vi "Compile Event Measure 1.1 Data.vi"(7 "RIO Address":string, 8 "error in (no error)":errorcluster, 11 "Device Item Ref in":T3 format="%.0x") -> (0 "error out":errorcluster, 2 "Event Timing Measures":T1[](array[typedef]), 3 "Device Item Ref out":T3 format="%.0x")   [LabVIEW 2015, in "Engine Simulation Toolkit System Explorer.lvlib"]
uses:
  Engine Simulation Toolkit System Explorer.lvlib
  <vilib>/NI Veristand/Custom Device API/Custom Device Item Ref.ctl
  Shared/1.1 Event Timing Measure Engine Data.ctl
  Shared/1.0 Event Timing Measure FIFO Idxs.ctl
  Polarity.ctl
  Shared/Constants and GUIDs.vi
  <vilib>/NI Veristand/Custom Device Tools/Custom Device Utility Library/NI VeriStand - Search for All Items by GUID.vi
  Shared/Engine Simulation Toolkit Shared.lvlib
  <vilib>/NI VeriStand/Custom Device Tools/Custom Device Utility Library/Custom Device Utility Library.lvlib
  <vilib>/NI VeriStand/Custom Device API/Custom Device API.lvlib
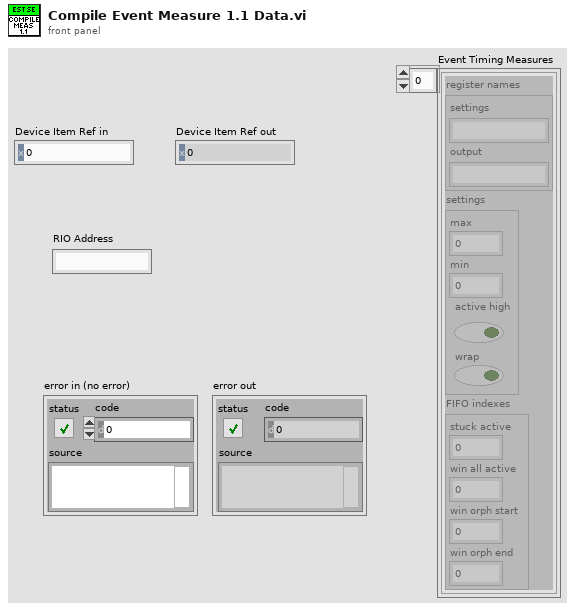
[diagram p1: front panel]
types:
  T1 = typedef "Engine Simulation Toolkit Shared.lvlib/1.1 Event Timing Measure Engine Data.ctl" = cluster{"register names":cluster{"settings":string, "output":string}, "settings":cluster{"max":u16, "min":u16, "active high":bool, "wrap":bool}, "FIFO indexes":T2}
  T2 = typedef "Engine Simulation Toolkit Shared.lvlib/1.0 Event Timing Measure FIFO Idxs.ctl" = cluster{"stuck active":i32, "win all active":i32, "win orph start":i32, "win orph end":i32}
  T3 = typedef "Custom Device API.lvlib/Custom Device Item Ref.ctl" = u64
  T4 = typedef "Engine Simulation Toolkit Shared.lvlib/Channel.ctl" = cluster{"Name":string, "Units":string, "Default":dbl, "Description":string, "Scalable":bool}
  T5 = typedef "Custom Device API.lvlib/Custom Device Item Info.ctl" = cluster{"Name":string, "Is Channel":bool, "GUID":string, "Is Waveform":bool}
  T6 = typedef "Engine Simulation Toolkit System Explorer.lvlib/Event Timing Window.ctl" = cluster{"Name":string, "Min":dbl, "Max":dbl, "Ref":dbl}
  T7 = typedef "Engine Simulation Toolkit System Explorer.lvlib/Event Timing Measurement.ctl" = cluster{"Name":string, "Bitfile name":string, "Window":string, "Polarity":T8}
  T8 = typedef "Engine Simulation Toolkit System Explorer.lvlib/Polarity.ctl" = enum16{"Active low", "Active high"}
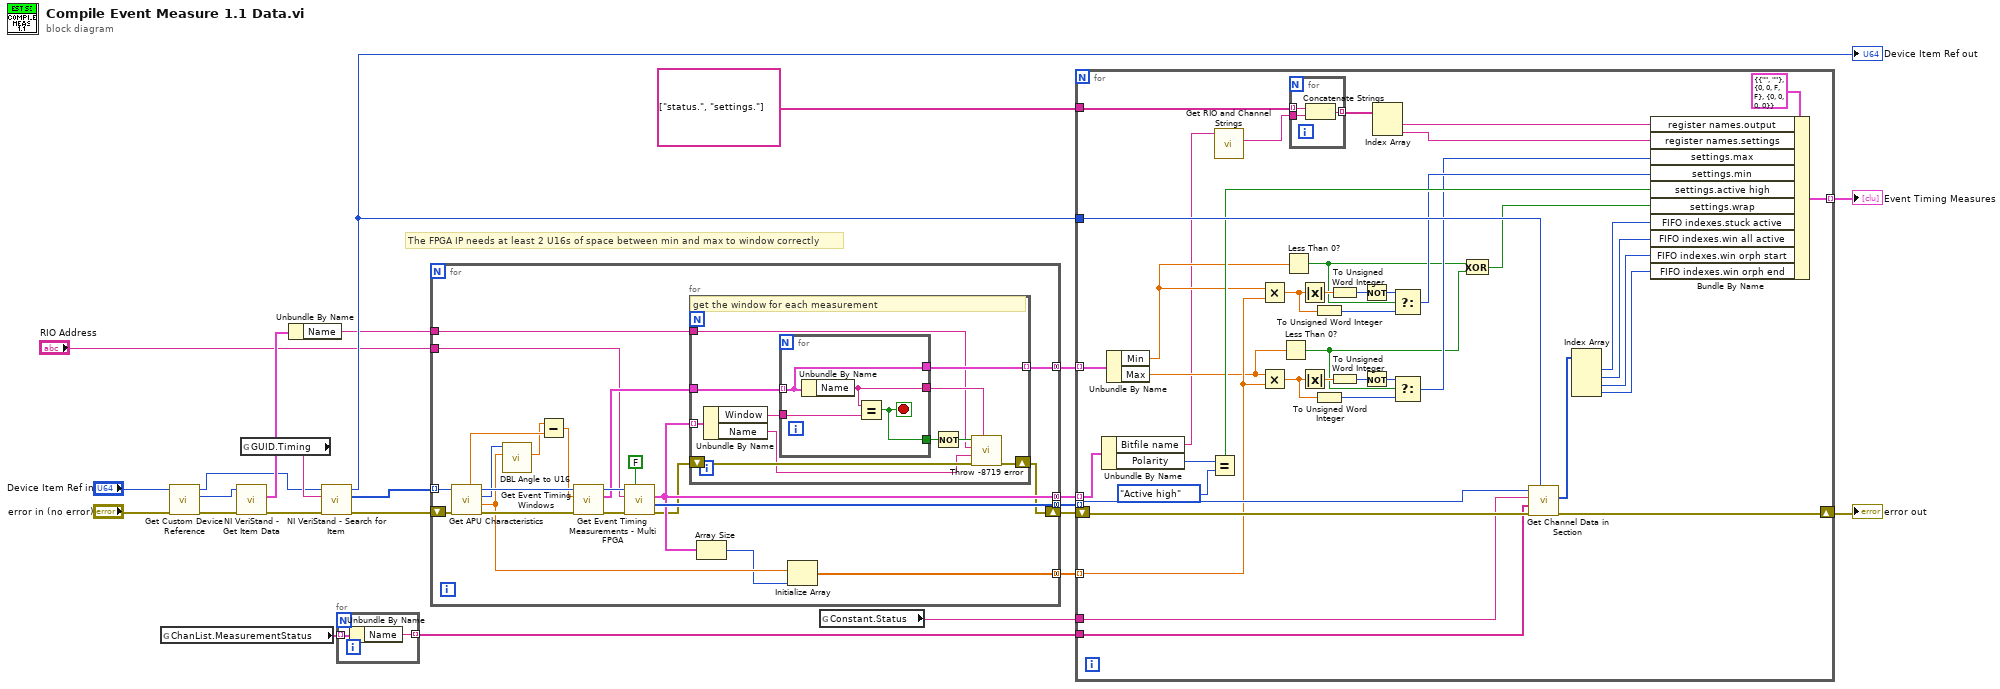
[diagram p0: block diagram]
diagram:
  # "The FPGA IP needs at least 2 U16s of space between min and max to window correctly"
  n1 = global read "Constants and GUIDs.vi" "ChanList.MeasurementStatus"() -> (w19:T4[])
  n2 = call "Get Custom Device Reference.vi"("error in (no error)"="error in (no error)", "Item Ref in"="Device Item Ref in") -> ("error out"=w5:errorcluster, "Custom Device Ref"=w2:T3, "Item Ref out"=w3:T3)  [unwired: 7 in]
  n3 = call <vilib>:"NI VeriStand - Get Item Data.vi"("error in (no error)"=w5, "Item Ref in"=w2) -> ("error out"=w9:errorcluster, "Item Info"=w8:T5)  [unwired: 6 in, 2 out]
  n4 = global read "Constants and GUIDs.vi" "GUID.Timing"() -> (w17:string)
  n5 = Unbundle By Name(w8) -> ("Name"=w7:string)
  n6 = call-poly <vilib>:"NI VeriStand - Search for Item.vi"("error in"=w9, "Item GUID"=w17, "Section Ref in"=w3) -> ("error out"=w24:errorcluster, "Item Refs"=w15:T3[], "Section Ref out"=w20:T3)  [unwired: 5 in, 1 out]
  "Device Item Ref out" <- w20
  n7 = for {
    tunnel: w19 -> [w26] mode=indexing
    tunnel: [w25] -> w18 mode=indexing
    n8 = Unbundle By Name(w26) -> ("Name"=w25:string)
  }
  n9 = for {
    tunnel: w15 -> [w43] mode=indexing
    shift-right: [w33] -> w16
    shift-left: w24 -> [w48]
    tunnel: [w39] -> w14 mode=concatenating
    tunnel: [w47] -> w13 mode=concatenating
    tunnel: [w40] -> w12 mode=concatenating
    tunnel: [w37] -> w11 mode=concatenating
    tunnel: w7 -> [w32]
    tunnel: "RIO Address" -> [w27]
    n10 = call "Get APU Characteristics.vi"("error in (no error)"=w48, "Item Ref in"=w43) -> ("error out"=w44:errorcluster, "angle to u16 scale factor"=w38:dbl, "total angle span (degrees)"=w35:u16, "Item Ref out"=w42:T3, "degrees of one u16"=w31:dbl)  [unwired: 3 in, 2 out]
    n11 = call "DBL Angle to U16.vi"("angle to u16 scale factor"=w38, "Desired angle (degrees)"=w35) -> ("Actual angle (degrees)"=w30:dbl)  [unwired: 8 in, 1 out]
    n12 = Subtract(x=w30, y=w31) -> (x-y=w29:dbl)
    n13 = call "Get Event Timing Windows.vi"("error in (no error)"=w44, "Max engine angle"=w29, "Item Ref in"=w42) -> ("error out"=w46:errorcluster, "Windows"=w41:T6[], "Item Ref out"=w45:T3)  [unwired: 6 in]
    n14 = call "Get Event Timing Measurements - Multi FPGA.vi"("return not-added measurements (T)"=FALSE, "error in (no error)"=w46, "RIO Address"=w27, "Item Ref in"=w45) -> ("error out"=w34:errorcluster, "measurements refs"=w47:T3[], "measurements"=w39:T7[])  [unwired: 3 in, 2 out]
    n15 = for {
      tunnel: w39 -> [w59] mode=indexing
      tunnel: w41 -> [w58]
      tunnel: [w56] -> w40 mode=indexing
      shift-right: [w52] -> w33
      shift-left: w34 -> [w51]
      tunnel: w32 -> [w49]
      # "get the window for each measurement"
      n16 = Unbundle By Name(w59) -> ("Window"=w57:string, "Name"=w50:string)
      n17 = for {
        tunnel: w58 -> [w62] mode=indexing
        tunnel: w57 -> [w63]
        tunnel: [w62] -> w56
        tunnel: [w61] -> w55
        tunnel: [w60] -> w53
        stop <- w61 stop-if-true
        n18 = Unbundle By Name(w62) -> ("Name"=w60:string)
        n19 = Equal?(x=w60, y=w63) -> (x = y?=w61:bool)
      }
      n20 = Not(x=w55) -> (.not. x?=w54:bool)
      n21 = call "Throw -8719 error.vi"("window name"=w53, "error in (no error)"=w51, "measurement name"=w50, "Custom device name"=w49, "Error"=w54) -> ("error out"=w52:errorcluster)  [unwired: 6 in]
    }
    n22 = Array Size(array=w39) -> (size(s)=w36:i32)
    n23 = Initialize Array(w38, w36) -> (w37:dbl[])
  }
  n24 = global read "Constants and GUIDs.vi" "Constant.Status"() -> (w10:string)
  n25 = for {
    shift-right: [w98] -> w22
    shift-left: w16 -> [w101]
    tunnel: string[] ["status.", "settings."] -> [w105]
    tunnel: w18 -> [w99]
    tunnel: [w103] -> w21 mode=indexing
    tunnel: w20 -> [w100]
    tunnel: w14 -> [w89] mode=indexing
    tunnel: w13 -> [w78] mode=indexing
    tunnel: w12 -> [w90] mode=indexing
    tunnel: w11 -> [w72] mode=indexing
    tunnel: w10 -> [w77]
    n26 = Unbundle By Name(w89) -> ("Bitfile name"=w65:string, "Polarity"=w88:T8)
    n27 = Unbundle By Name(w90) -> ("Min"=w80:dbl, "Max"=w69:dbl)
    n28 = Equal?(x=w88, y=Polarity."Active high") -> (x = y?=w86:bool)
    n29 = call "Get RIO and Channel Strings.vi"("rio/channel"=w65) -> ("channel"=w64:string)  [unwired: 9 in, 1 out]
    n30 = Multiply(x=w80, y=w72) -> (x*y=w81:dbl)
    n31 = Multiply(x=w69, y=w72) -> (x*y=w70:dbl)
    n32 = Less Than 0?(x=w69) -> (x < 0?=w67:bool)
    n33 = Less Than 0?(x=w80) -> (x < 0?=w68:bool)
    n34 = for {
      tunnel: w105 -> [w108] mode=indexing
      tunnel: [w107] -> w102 mode=indexing
      tunnel: w64 -> [w106]
      n35 = Concatenate Strings(w108, w106) -> (w107:string)
    }
    n36 = Absolute Value(x=w81) -> (abs(x)=w83:dbl)
    n37 = Absolute Value(x=w70) -> (abs(x)=w75:dbl)
    n38 = To Unsigned Word Integer(number=w81) -> (unsigned 16bit integer=w85:u16)
    n39 = To Unsigned Word Integer(number=w70) -> (unsigned 16bit integer=w73:u16)
    n40 = To Unsigned Word Integer(number=w83) -> (unsigned 16bit integer=w82:u16)
    n41 = To Unsigned Word Integer(number=w75) -> (unsigned 16bit integer=w76:u16)
    n42 = Not(x=w82) -> (.not. x?=w84:u16)
    n43 = Not(x=w76) -> (.not. x?=w74:u16)
    n44 = Index Array(array=w102) -> (element #1=w96:string, element #2=w95:string)  [unwired: 2 in]
    n45 = Select(t=w84, s=w68, f=w85) -> (s? t:f=w79:u16)
    n46 = Select(t=w74, s=w67, f=w73) -> (s? t:f=w71:u16)
    n47 = Exclusive Or(1:w67, 2:w68) -> (0:w66:bool)
    n48 = call "Get Channel Data in Section.vi"("Custom device ref"=w100, "error in (no error)"=w101, "Channels"=w99, "Section (\"\":none)"=w77, "Item Ref in"=w78) -> ("error out"=w98:errorcluster, "FIFO indexes"=w97:i32[])  [unwired: 2 in, 3 out]
    n49 = Index Array(array=w97) -> (element #1=w94:i32, element #2=w93:i32, element #3=w92:i32, element #4=w91:i32)  [unwired: 4 in]
    n50 = Bundle By Name(cluster=T1 {"register names"={"settings"="", "output"=""}, "settings"={"max"=0, "min"=0, "active high"=FALSE, "wrap"=FALSE}, "FIFO indexes"={"stuck active"=0, "win all active"=0, "win orph start"=0, "win orph end"=0}} ("1.0.0 Event Timing Measure"), "register names.output"=w96, "register names.settings"=w95, "settings.max"=w71, "settings.min"=w79, "settings.active high"=w86, "settings.wrap"=w66, "FIFO indexes.stuck active"=w94, "FIFO indexes.win all active"=w93, "FIFO indexes.win orph start"=w92, "FIFO indexes.win orph end"=w91) -> (w103:T1)
  }
  "error out" <- w22
  "Event Timing Measures" <- w21
